vi "GV line clock.vi"() -> ()   [LabVIEW 2017]
panel:
  in  "Line clock":bool
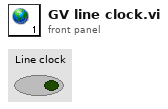
[diagram p1: front panel]
diagram:
